vi "session_set_one_property_boolean.vi"(6 "Skip setting if in Options string (F)":bool, 7 "Session Parameter Boolean":T1, 8 "error in":errorcluster caption="error in (no error)", 10 "Boolean value in":bool, 11 "VISA resource name":refnum<visa-resource-name>) -> (0 "error out":errorcluster, 2 "Set in the Options string":bool, 3 "VISA resource name out":refnum<visa-resource-name>)   [LabVIEW 2022 SP3, in "hmp4000_rsidr_core.lvlib"]
uses:
  hmp4000_rsidr_core.lvlib
  type_Session_Parameter_Boolean.ctl
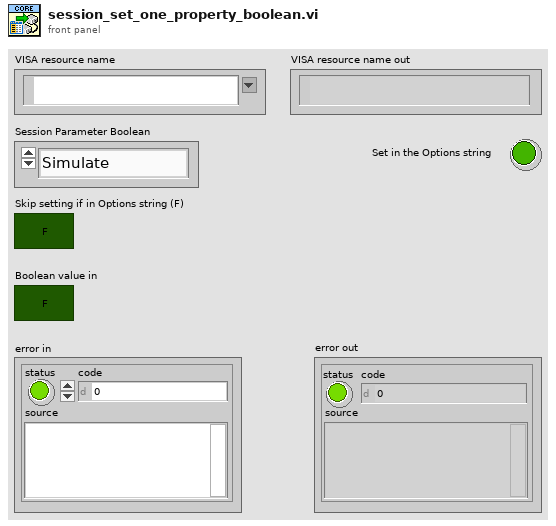
[diagram p1: front panel]
types:
  T1 = typedef "hmp4000_rsidr_core.lvlib/type_Session_Parameter_Boolean.ctl" = enum16{"Simulate", "Query Instr Status", "Check Range", "Check Options", "Add LF to Write", "Duplicate Session", "Fast Sweep", "Logging"}
  T2 = typedef "hmp4000_rsidr_core.lvlib/type_Session_Data.ctl" = cluster{"IDN string":string, "Instrument FW":string, "Instr type":string, "Instr type for err. msg.":string, "Installed Options":string[], "Ignore Error Messages":string, "Logging params":variant, "OPC Timeout":i32, "VISA Timeout":i32, "STB Poll VISA Timeout":i32, "Additional Flags":i32, "Wait Before Read":i32, "Wait Before Write":i32, "Option String Flags":i32, "IO Segment Size":i64, "VISA Access Mode":T3, "Interface Type":T4, "OPC Wait Mode":T5, "Bin Float Number  Format":T6, "Bin Integer Number Format":T7, "Simulate":bool, "VXIcapable":bool, "Duplicate Session":bool, "Add LF to Write":bool, "Logging":bool, "Fast Sweep":bool, "Query Instrument Status":bool, "Check Range":bool, "Check Options":bool}
  T3 = typedef "hmp4000_rsidr_core.lvlib/type_VisaAccessMode.ctl" = u16
  T4 = typedef "hmp4000_rsidr_core.lvlib/type_InterfaceType.ctl" = enum16{"Unknown", "GPIB", "VXI", "GPIB_VXI", "ASRL", "PXI", "TCPIP", "USB", "SOCKET"}
  T5 = typedef "hmp4000_rsidr_core.lvlib/type_OPC_Wait_Mode.ctl" = enum16{"STBpolling", "STBpollingSlow", "STBpollingSuperSlow", "ServiceRequest", "OPCquery"}
  T6 = typedef "hmp4000_rsidr_core.lvlib/type_Binary_Float_Number_Format.ctl" = enum16{"Float_4_Bytes_Swapped", "Float_4_Bytes", "Double_8_Bytes_Swapped", "Double_8_Bytes"}
  T7 = typedef "hmp4000_rsidr_core.lvlib/type_Binary_Integer_Number_Format.ctl" = enum16{"Int32_4_Bytes_Swapped", "Int32_4 Bytes", "Int16_2_Bytes_Swapped", "Int16_2_Bytes"}
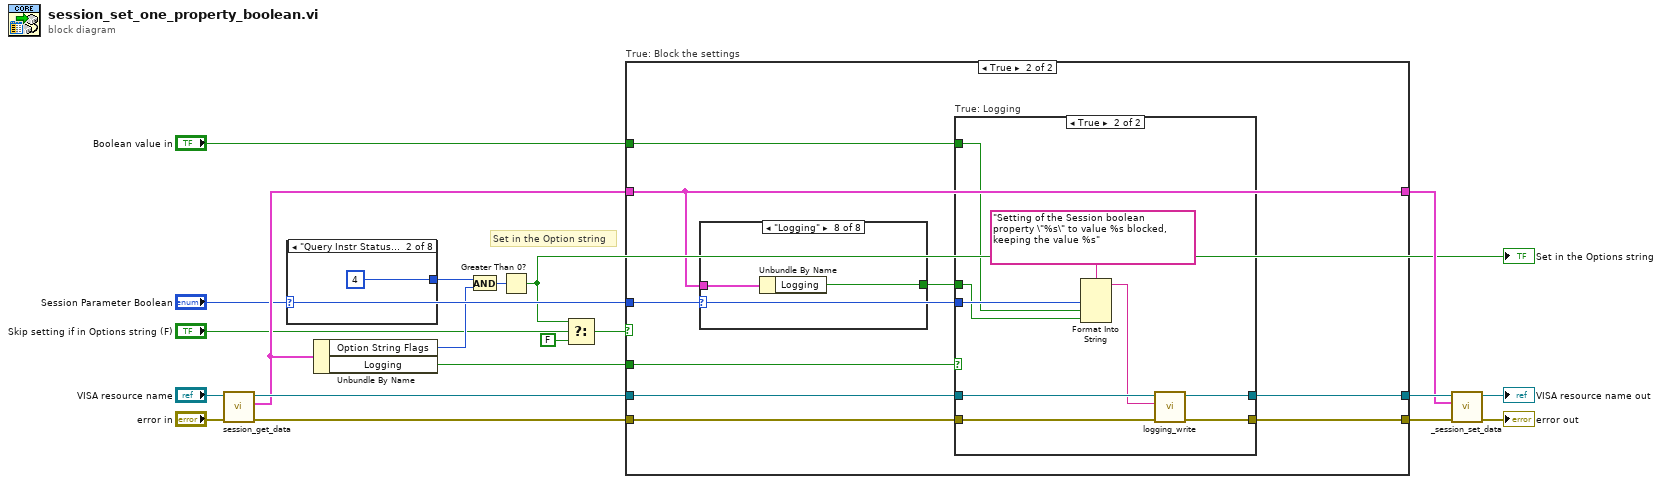
[diagram p0: block diagram]
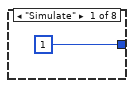
[diagram p2: hidden frame]
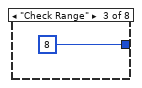
[diagram p3: hidden frame]
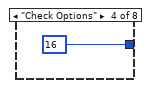
[diagram p4: hidden frame]
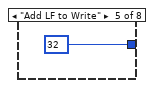
[diagram p5: hidden frame]
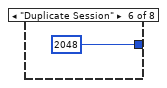
[diagram p6: hidden frame]
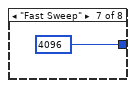
[diagram p7: hidden frame]
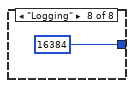
[diagram p8: hidden frame]
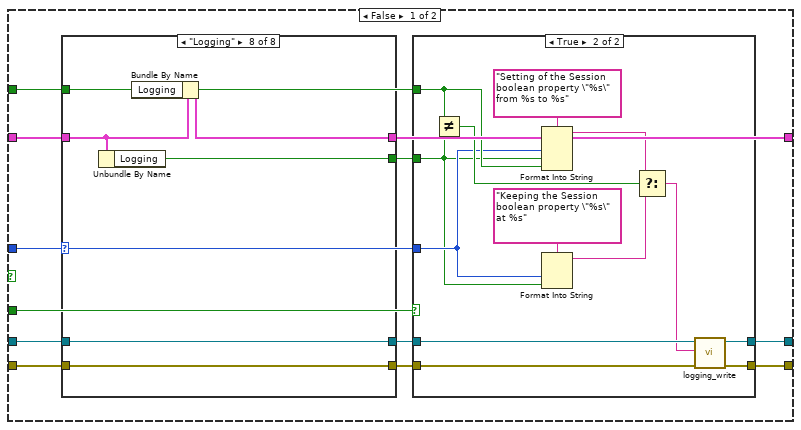
[diagram p9: hidden frame]
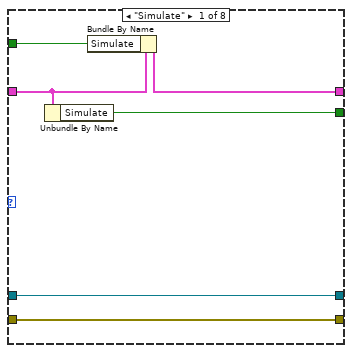
[diagram p11: hidden frame]
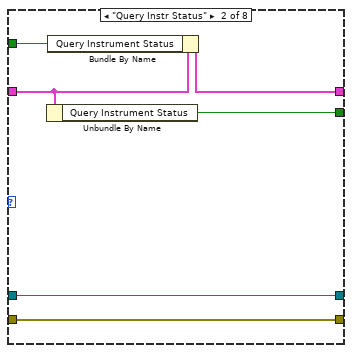
[diagram p12: hidden frame]
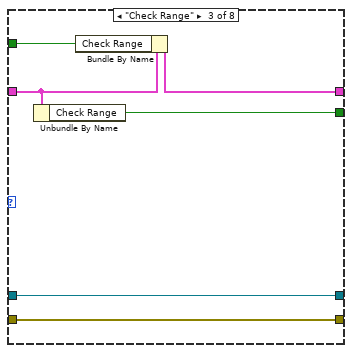
[diagram p13: hidden frame]
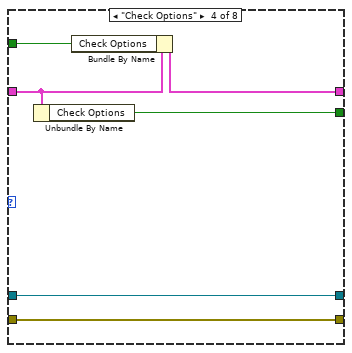
[diagram p14: hidden frame]
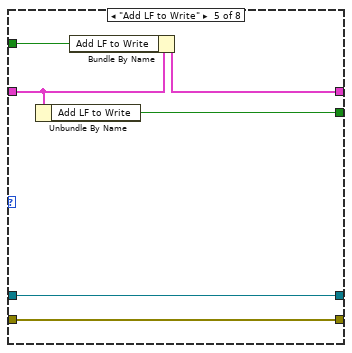
[diagram p15: hidden frame]
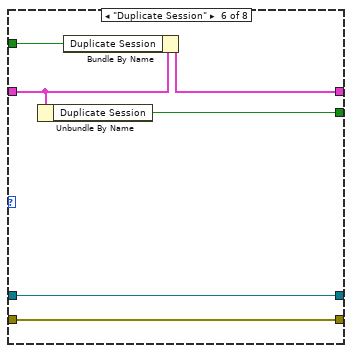
[diagram p16: hidden frame]
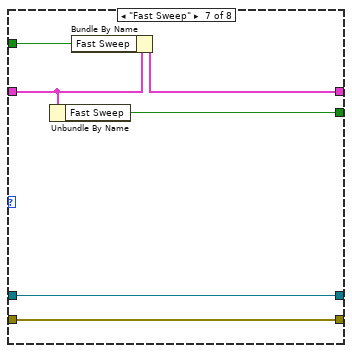
[diagram p17: hidden frame]
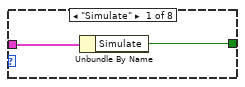
[diagram p18: hidden frame]
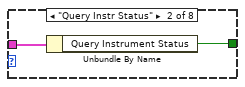
[diagram p19: hidden frame]
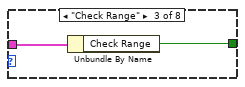
[diagram p20: hidden frame]
diagram:
  # "Set in the Option string"
  n1 = call "session_get_data.vi"("error in"="error in", "VISA resource name"="VISA resource name") -> ("error out"=w17:errorcluster, "Session User Data out"=w11:T2, "VISA resource name out"=w16:refnum<visa-resource-name>)  [unwired: 6 in, 1 out]
  n2 = case shown="\"Query Instr Status\"" "Session Parameter Boolean" {
    tunnel: [1 4 8 16 32 2048 4096 16384] -> w7
    frame "Simulate" {
    }
    frame "Query Instr Status" {
    }
    frame "Check Range" {
    }
    frame "Check Options" {
    }
    frame "Add LF to Write" {
    }
    frame "Duplicate Session" {
    }
    frame "Fast Sweep" {
    }
    frame "Logging" {
    }
  }
  n3 = Unbundle By Name(w11) -> ("Option String Flags"=w6:i32, "Logging"=w8:bool)
  n4 = And(x=w7, y=w6) -> (x .and. y?=w4:i32)
  n5 = Greater Than 0?(x=w4) -> (x > 0?=w2:bool)
  "Set in the Options string" <- w2
  n6 = Select(t=w2, s="Skip setting if in Options string (F)", f=FALSE) -> (s? t:f=w3:bool)
  n7 = case "True: Block the settings" shown="True" w3 {
    tunnel: "Session Parameter Boolean" -> [w33 w106]
    tunnel: w11 -> [w40 w105]
    tunnel: "Boolean value in" -> [w35 w107]
    tunnel: [w39 w105] -> w10
    tunnel: w17 -> [w38 w111]
    tunnel: w16 -> [w37 w110]
    tunnel: [w30 w109] -> w15
    tunnel: [w29 w108] -> w14
    tunnel: w8 -> [w34 w112]
    frame False {
      n8 = case shown="\"Logging\"" w33 {
        tunnel: w35 -> [w61 w67 w73 w79 w85 w91 w97 w103]
        tunnel: w40 -> [w57 w63 w69 w75 w81 w87 w93 w99]
        tunnel: [w58 w64 w70 w76 w82 w88 w94 w100] -> w39
        tunnel: w38 -> [w59 w66 w72 w78 w84 w90 w95 w101]
        tunnel: w37 -> [w60 w65 w71 w77 w83 w89 w96 w102]
        tunnel: [w59 w66 w72 w78 w84 w90 w95 w101] -> w32
        tunnel: [w60 w65 w71 w77 w83 w89 w96 w102] -> w31
        tunnel: [w56 w62 w68 w74 w80 w86 w92 w98] -> w36
        frame "Simulate" {
          n9 = Unbundle By Name(w57) -> ("Simulate"=w56:bool)
          n10 = Bundle By Name(cluster=w57, "Simulate"=w61) -> (w58:T2)
        }
        frame "Query Instr Status" {
          n11 = Unbundle By Name(w63) -> ("Query Instrument Status"=w62:bool)
          n12 = Bundle By Name(cluster=w63, "Query Instrument Status"=w67) -> (w64:T2)
        }
        frame "Check Range" {
          n13 = Unbundle By Name(w69) -> ("Check Range"=w68:bool)
          n14 = Bundle By Name(cluster=w69, "Check Range"=w73) -> (w70:T2)
        }
        frame "Check Options" {
          n15 = Unbundle By Name(w75) -> ("Check Options"=w74:bool)
          n16 = Bundle By Name(cluster=w75, "Check Options"=w79) -> (w76:T2)
        }
        frame "Add LF to Write" {
          n17 = Unbundle By Name(w81) -> ("Add LF to Write"=w80:bool)
          n18 = Bundle By Name(cluster=w81, "Add LF to Write"=w85) -> (w82:T2)
        }
        frame "Duplicate Session" {
          n19 = Unbundle By Name(w87) -> ("Duplicate Session"=w86:bool)
          n20 = Bundle By Name(cluster=w87, "Duplicate Session"=w91) -> (w88:T2)
        }
        frame "Fast Sweep" {
          n21 = Unbundle By Name(w93) -> ("Fast Sweep"=w92:bool)
          n22 = Bundle By Name(cluster=w93, "Fast Sweep"=w97) -> (w94:T2)
        }
        frame "Logging" {
          n23 = Unbundle By Name(w99) -> ("Logging"=w98:bool)
          n24 = Bundle By Name(cluster=w99, "Logging"=w103) -> (w100:T2)
        }
      }
      n25 = case shown="True" w34 {
        tunnel: w36 -> [_ w43]
        tunnel: w35 -> [_ w45]
        tunnel: w33 -> [_ w44]
        tunnel: w32 -> [w41 w51]
        tunnel: w31 -> [w42 w50]
        tunnel: [w41 w49] -> w30
        tunnel: [w42 w48] -> w29
        frame False {
        }
        frame True {
          n26 = Not Equal?(x=w45, y=w43) -> (x != y?=w46:bool)
          n27 = Format Into String(format string="Setting of the Session boolean property \"%s\" from %s to %s", w44, w43, w45) -> (resulting string=w54:string)  [unwired: 2 in, 1 out]
          n28 = Format Into String(format string="Keeping the Session boolean property \"%s\" at %s", w44, w43) -> (resulting string=w55:string)  [unwired: 2 in, 1 out]
          n29 = Select(t=w54, s=w46, f=w55) -> (s? t:f=w47:string)
          n30 = call "logging_write.vi"("error in"=w51, "String to write"=w47, "VISA resource name"=w50) -> ("error out"=w49:errorcluster, "VISA resource name out"=w48:refnum<visa-resource-name>)  [unwired: 7 in]
        }
      }
    }
    frame True {
      n31 = case shown="\"Logging\"" w106 {
        tunnel: w105 -> [w114 w116 w118 w120 w122 w124 w126 w128]
        tunnel: [w113 w115 w117 w119 w121 w123 w125 w127] -> w104
        frame "Simulate" {
          n32 = Unbundle By Name(w114) -> ("Simulate"=w113:bool)
        }
        frame "Query Instr Status" {
          n33 = Unbundle By Name(w116) -> ("Query Instrument Status"=w115:bool)
        }
        frame "Check Range" {
          n34 = Unbundle By Name(w118) -> ("Check Range"=w117:bool)
        }
        frame "Check Options" {
          n35 = Unbundle By Name(w120) -> ("Check Options"=w119:bool)
        }
        frame "Add LF to Write" {
          n36 = Unbundle By Name(w122) -> ("Add LF to Write"=w121:bool)
        }
        frame "Duplicate Session" {
          n37 = Unbundle By Name(w124) -> ("Duplicate Session"=w123:bool)
        }
        frame "Fast Sweep" {
          n38 = Unbundle By Name(w126) -> ("Fast Sweep"=w125:bool)
        }
        frame "Logging" {
          n39 = Unbundle By Name(w128) -> ("Logging"=w127:bool)
        }
      }
      n40 = case "True: Logging" shown="True" w112 {
        tunnel: w111 -> [w130 w139]
        tunnel: w110 -> [w129 w138]
        tunnel: [w130 w137] -> w109
        tunnel: [w129 w136] -> w108
        tunnel: w106 -> [_ w135]
        tunnel: w107 -> [_ w132]
        tunnel: w104 -> [_ w131]
        frame False {
        }
        frame True {
          n41 = Format Into String(format string="Setting of the Session boolean property \"%s\" to value %s blocked, keeping the value %s", w135, w132, w131) -> (resulting string=w133:string)  [unwired: 2 in, 1 out]
          n42 = call "logging_write.vi"("error in"=w139, "String to write"=w133, "VISA resource name"=w138) -> ("error out"=w137:errorcluster, "VISA resource name out"=w136:refnum<visa-resource-name>)  [unwired: 7 in]
        }
      }
    }
  }
  n43 = call "_session_set_data.vi"("error in"=w15, "Session User Data in"=w10, "VISA resource name"=w14) -> ("error out"=→"error out":errorcluster, "VISA resource name out"=→"VISA resource name out":refnum<visa-resource-name>)  [unwired: 7 in]
